vi "设置加工方法（简单工厂）.vi"(8 "error in (no error)":errorcluster caption="错误输入（无错误）", 10 "加工方法":T1, 11 "加工中心 输入":refnum<class "加工中心.lvclass"> caption="DNL_LabVIEW Object in") -> (0 "error out":errorcluster caption="错误输出", 3 "加工中心 输出":refnum<class "加工中心.lvclass"> caption="DNL_LabVIEW Object out")   [LabVIEW 2011, in "加工中心.lvclass"]
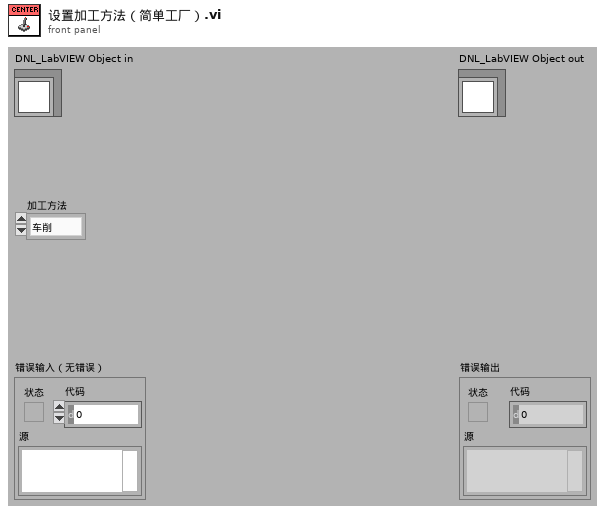
[diagram p1: front panel]
types:
  T1 = typedef "简单加工类工厂.lvclass/加工方法.ctl" = enum16{"车削", "铣削", "钻削"}
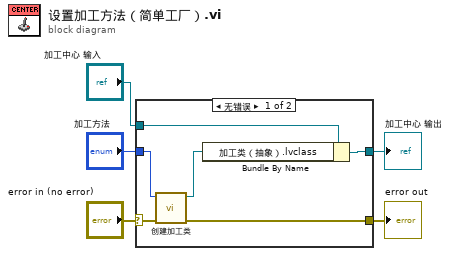
[diagram p0: block diagram]
diagram:
  n1 = case shown="无错误" "error in (no error)" {
    selector: "error in (no error)" -> [w10 w13]
    tunnel: [w9 w13] -> w4
    tunnel: [w7 w12] -> w2
    tunnel: "加工中心 输入" -> [w8 w12]
    tunnel: "加工方法" -> [w11 _]
    frame No Error {
      n2 = call "创建加工类.vi"("error in (no error)"=w10, "加工方法"=w11) -> ("error out"=w9:errorcluster, "加工类（抽象）.lvclass"=w6:refnum<class "加工类（抽象）.lvclass">)  [unwired: 8 in]
      n3 = Bundle By Name(cluster=w8, "加工类（抽象）.lvclass"=w6) -> (w7:refnum<class "加工中心.lvclass">)
    }
    frame Error {
    }
  }
  "error out" <- w4
  "加工中心 输出" <- w2
